vi "Read Oxygen Temperature.vi"(0 "Session Handle in":T2, 5 "Temperature Sensors":T1=51 items=["TS1"=51, "TS2"=52, "TS3"=53], 11 "error in (no error)":errorcluster) -> (4 "Session Handle out":T2, 6 "Temperature":dbl, 15 "error out":errorcluster)   [LabVIEW 2015, in "Gas.lvclass"]
uses:
  Gas.lvclass
  Typedefs/Session Handle.ctl
  Typedefs/Temperature Sensors.ctl
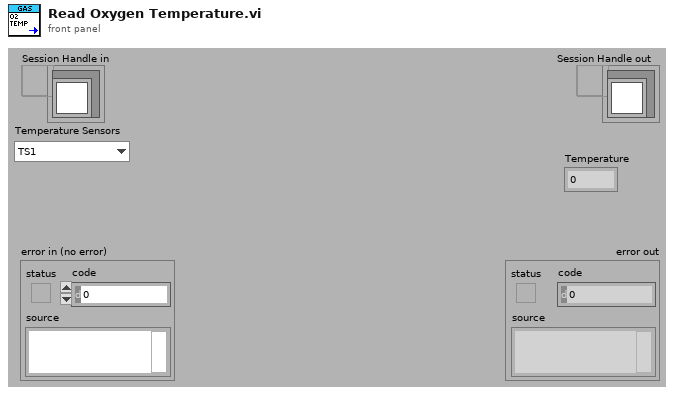
[diagram p1: front panel]
types:
  T1 = typedef "Gas.lvclass/Temperature Sensors.ctl" = u16
  T2 = typedef "Gas.lvclass/Session Handle.ctl" = refnum<data-value>
  T3 = typedef "XNET Frame CAN.ctl" = cluster{"timestamp":timestamp, "payload":u8[], "identifier":u32, "type":T4, "extended?":bool, "echo?":bool}
  T4 = typedef "XNET Frame Type CAN.ctl" = u8
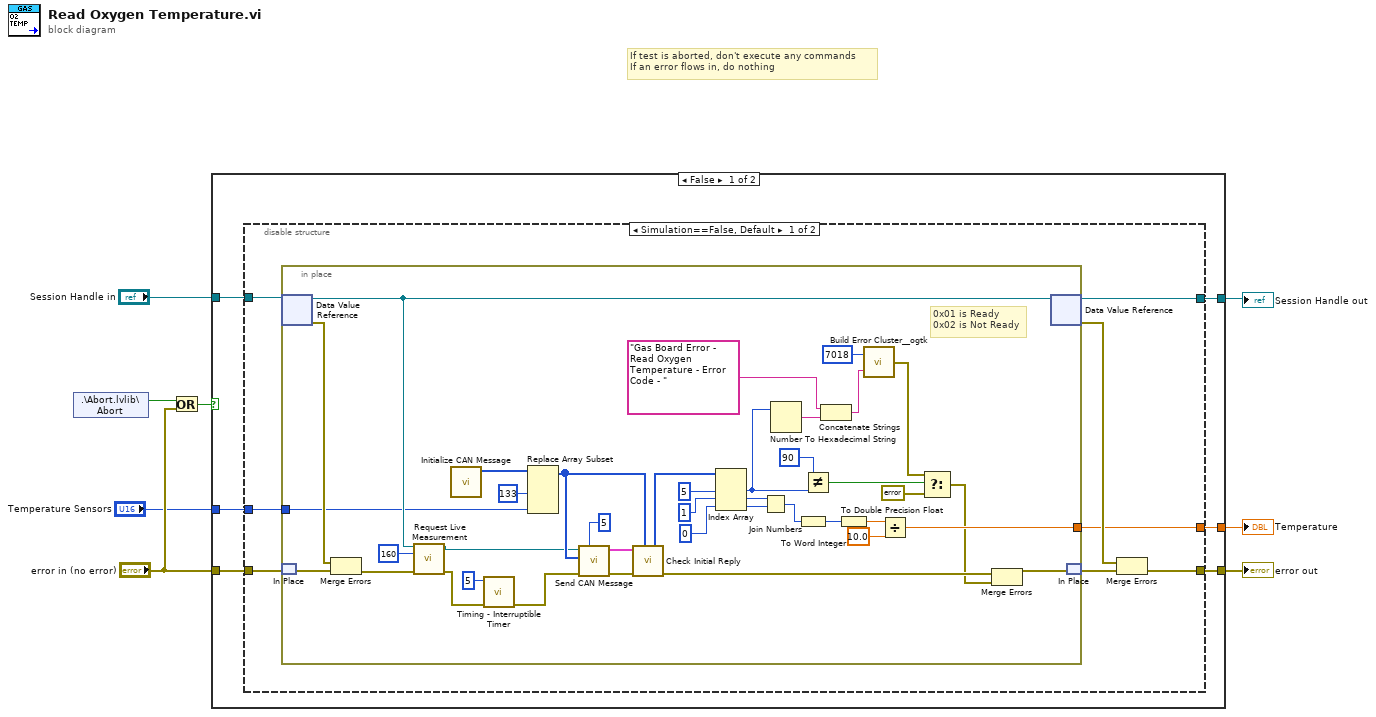
[diagram p0: block diagram]
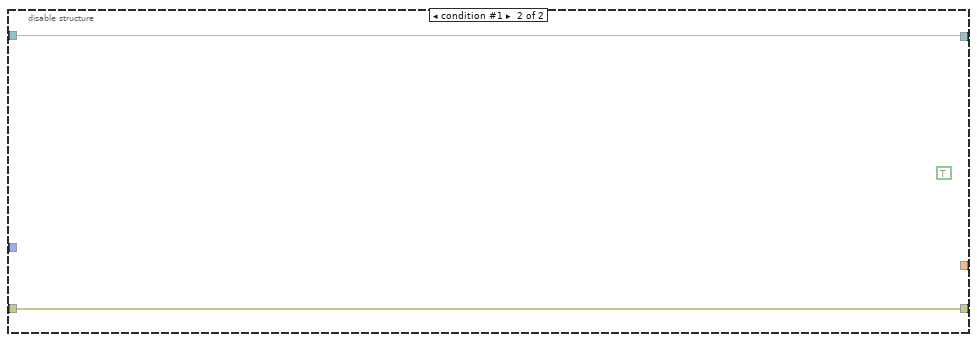
[diagram p2: hidden frame]
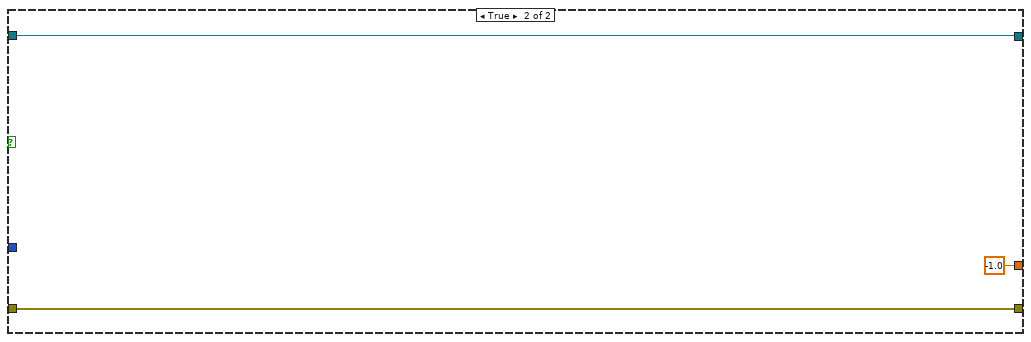
[diagram p3: hidden frame]
diagram:
  # "If test is aborted, don't execute any commands\nIf an error flows in, do nothing"
  n1 = shared-variable ".\\Abort.lvlib\\Abort"() -> (w5:bool)  [unwired: 1 in, 1 out]
  n2 = Or(x=w5, y="error in (no error)") -> (x .or. y?=w3:bool)
  n3 = case shown="False" w3 {
    tunnel: [w14 w66] -> w7
    tunnel: [w13 w65] -> w6
    tunnel: "Session Handle in" -> [w12 w66]
    tunnel: "error in (no error)" -> [w11 w65]
    tunnel: "Temperature Sensors" -> [w10 _]
    tunnel: [w9 -1.0] -> w1
    frame False {
      n4 = disable-structure shown="Simulation==False, Default" {
        disable-tunnel: [w22 w63] -> w14
        disable-tunnel: [w19 w62] -> w13
        disable-tunnel: w12 -> [w18 w63]
        disable-tunnel: w11 -> [w17 w62]
        disable-tunnel: w10 -> [w16 _]
        disable-tunnel: [w15 _] -> w9
        frame condition #0 (active) {
          n5 = in-place {
            in-place-border: w16 -> [w38]
            in-place-border: [w30] -> w15
            # "0x01 is Ready\n0x02 is Not Ready"
            n6 = in-place-dvr #1(w18) -> (w40:refnum<class "Gas.lvclass">, w57:errorcluster)
            n7 = in-place-match #2(w17) -> (w56:errorcluster)
            n8 = Merge Errors(w57, w56) -> (w41:errorcluster)
            n9 = call "Request Live Measurement.vi"("Gas In"=w40, "Request Type"=u8 160, "error in (no error)"=w41) -> ("Gas Out"=w26:refnum<class "Gas.lvclass">, "error out"=w28:errorcluster)  [unwired: 10 in, 1 out]
            n10 = call "Initialize CAN Message.vi"() -> ("Initial Payload"=w59:u8[])  [unwired: 11 in]
            n11 = call "Timing - Interruptible Timer.vi"("error in (no error)"=w28, "Wait (s)"=5) -> ("error out"=w39:errorcluster)  [unwired: 7 in, 2 out]
            n12 = Replace Array Subset(array=w59, new element #1=u8 133 ("new element/subarray"), new element #2=w38) -> (w55:u8[])  [unwired: 2 in]
            n13 = call "Send CAN Message.vi"("Number of Retries"=5, "error in (no error)"=w39, "payload"=w55, "Gas In"=w26) -> ("error out"=w25:errorcluster, "Reply"=w53:T3[])  [unwired: 5 in, 1 out]
            n14 = call "Check Initial Reply.vi"("Write Message"=w55, "error in (no error)"=w25, "Reply"=w53) -> ("error out"=w24:errorcluster, "Data Packet"=w58:u8[])  [unwired: 5 in, 2 out]
            n15 = Index Array(array=w58, index #1=5 ("index"), index #2=1 ("index"), index #3=0 ("index")) -> (element #1=w46:u8, element #2=w36:u8, element #3=w35:u8)
            n16 = Join Numbers(hi=w36, lo=w35) -> ((hi.lo)=w33:u16)
            n17 = Number To Hexadecimal String(2:w46) -> (0:w44:string)  [unwired: 1 in]
            n18 = To Word Integer(number=w33) -> (16bit integer=w34:i16)
            n19 = Not Equal?(x=u8 90 ("new element/subarray"), y=w46) -> (x != y?=w49:bool)
            n20 = Concatenate Strings("Gas Board Error - Read Oxygen Temperature - Error Code - " ("string"), w44) -> (w42:string)
            n21 = To Double Precision Float(number=w34) -> (double precision float=w32:dbl)
            n22 = call <userlib>:"Build Error Cluster__ogtk.vi"("String to Prepend to source (\"\")"=w42, "code"=7018) -> ("error out"=w51:errorcluster)
            n23 = Divide(x=w32, y=10.0) -> (x/y=w30:dbl)
            n24 = Select(t=w51, s=w49, f=errorcluster {"status"=FALSE, "code"=0, "source"=""}) -> (s? t:f=w23:errorcluster)
            n25 = Merge Errors(w24, w23) -> (w60:errorcluster)
            n26 = in-place-dvr #1(w40) -> (w22:T2, w20:errorcluster)
            n27 = in-place-match #2(w60) -> (w21:errorcluster)
          }
          n28 = Merge Errors(w20, w21) -> (w19:errorcluster)
        }
        frame condition #1 {
          (unwired) TRUE
        }
      }
    }
    frame True {
    }
  }
  "Session Handle out" <- w7
  "error out" <- w6
  "Temperature" <- w1
